vi "List to 3D Array.vi"(8 "#Readings(0)":u16, 9 "#Channels(0)":u16, 10 "#Fields per Read (1)":u16=1, 11 "List(empty)":string) -> (2 "Output Array":dbl[][][](array[numeric]) format="%.2f")   [LabVIEW 2016, in "Agilent 34970.lvlib"]
doc: "Given a List of strings separated by commas, this VI returns a 3D array of numbers whose dimensions are F by C by R, where \n \nF is the number of fields per reading, \nC is the number of channels being read, \nR is the total number of readings (not per channel)\n\nThis VI is useful for charting values read from the instrument in comma-delimited form."
uses:
  Agilent 34970.lvlib
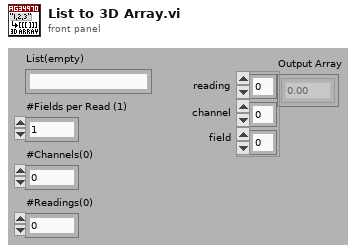
[diagram p1: front panel]
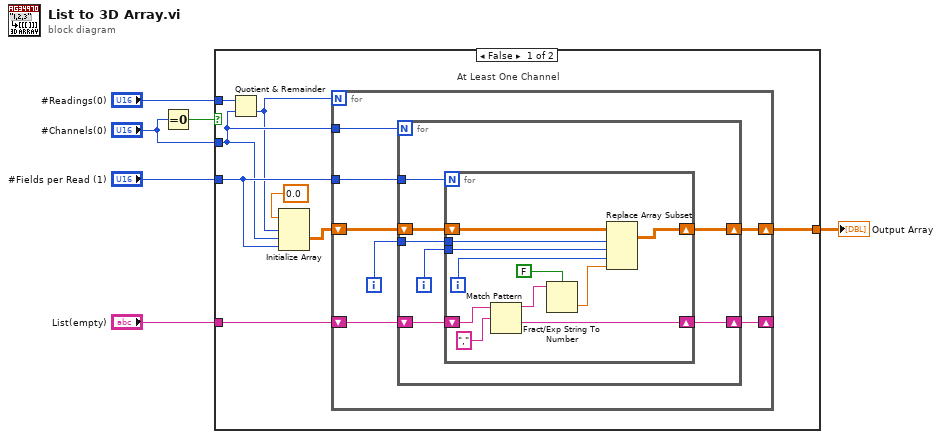
[diagram p0: block diagram]
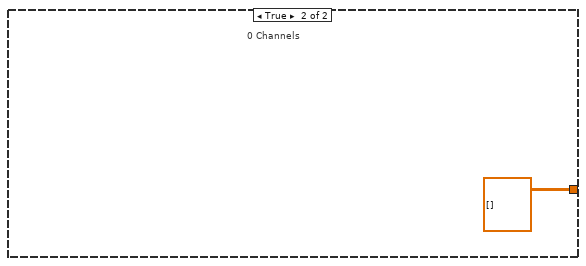
[diagram p2: hidden frame]
diagram:
  n1 = Equal To 0?(x="#Channels(0)") -> (x = 0?=w2:bool)
  n2 = case shown="False" w2 {
    tunnel: [w14 dbl[][][] []] -> w1
    tunnel: "#Readings(0)" -> [w9 _]
    tunnel: "#Channels(0)" -> [w8 _]
    tunnel: "List(empty)" -> [w12 _]
    tunnel: "#Fields per Read (1)" -> [w10 _]
    frame False {
      # "At Least One Channel"
      n3 = Quotient & Remainder(x=w9, y=w8) -> (floor(x/y)=w7:u16)  [unwired: 1 out]
      n4 = Initialize Array(0.0, w7, w8, w10) -> (w13:dbl[][][])
      n5 = for {
        N: w7 -> [_]
        tunnel: w8 -> [w21]
        tunnel: w10 -> [w20]
        shift-right: [w19] -> _
        shift-left: w12 -> [w18]
        shift-right: [w15] -> w14
        shift-left: w13 -> [w16]
        i -> [w17]
        n6 = for {
          N: w21 -> [_]
          tunnel: w20 -> [w28]
          shift-right: [w27] -> w19
          shift-left: w18 -> [w26]
          tunnel: w17 -> [w24]
          shift-right: [w22] -> w15
          shift-left: w16 -> [w23]
          i -> [w25]
          n7 = for {
            N: w28 -> [_]
            shift-right: [w35] -> w27
            shift-left: w26 -> [w39]
            tunnel: w25 -> [w34]
            tunnel: w24 -> [w33]
            shift-right: [w30] -> w22
            shift-left: w23 -> [w31]
            i -> [w32]
            n8 = Match Pattern(string=w39, regular expression=",") -> (before substring=w37:string, after substring=w35:string)  [unwired: 1 in, 2 out]
            n9 = Fract/Exp String To Number(use system decimal point (T)=FALSE, string=w37) -> (number=w36:dbl)  [unwired: 2 in, 1 out]
            n10 = Replace Array Subset(array=w31, new element=w36, index (dim 0)=w33, index (dim 1)=w34, index (dim 2)=w32) -> (w30:dbl[][][])
          }
        }
      }
    }
    frame True {
      # "0 Channels"
    }
  }
  "Output Array" <- w1
